vi "LAb4gui.vi"() -> ()   [LabVIEW 2026]
uses:
  Control_Lab4.ctl
  <vilib>/Instr/_visa.llb/VISA Configure Serial Port (Instr).vi
  Serial - Settings.ctl
panel:
  in  "Serial Settings":T1={"baud rate"=115200, "data bits"=8, "parity"=enum."None", "stop bits"=10, "flow control"=0} {"flow control" items=["None"=0, "XON/XOFF"=1, "RTS/CTS"=2, "DTR/DSR"=4]; "stop bits" items=["1.0"=10, "1.5"=15, "2.0"=20]; "data bits" min=5 max=8 step=1; "baud rate" items=["75"=75, "110"=110, "134"=134, "150"=150, "300"=300, "600"=600, "1200"=1200, "1800"=1800, "2400"=2400, "4800"=4800, "7200"=7200, "9600"=9600, "14400"=14400, "19200"=19200, "28800"=28800, "38400"=38400, "56000"=56000, "57600"=57600, "115200"=115200, "128000"=128000, "230400"=230400]}
  in  "Detection Threshold":i32
  in  "stop":bool
  out "Last Command Sent":string
  out "ESP Response":string
  in  "Send Filters":bool
  in  "Blur":dbl(knob) scale=0.0..10.0
  in  "Minimum Area":i32
  in  "Reset Filters":bool
  out "Connected to ESP":bool
  in  "VISA resource name":refnum<visa-resource-name>
  in  "Display ON/OFF":bool
  in  "Get Status":bool
  in  "Identify":bool
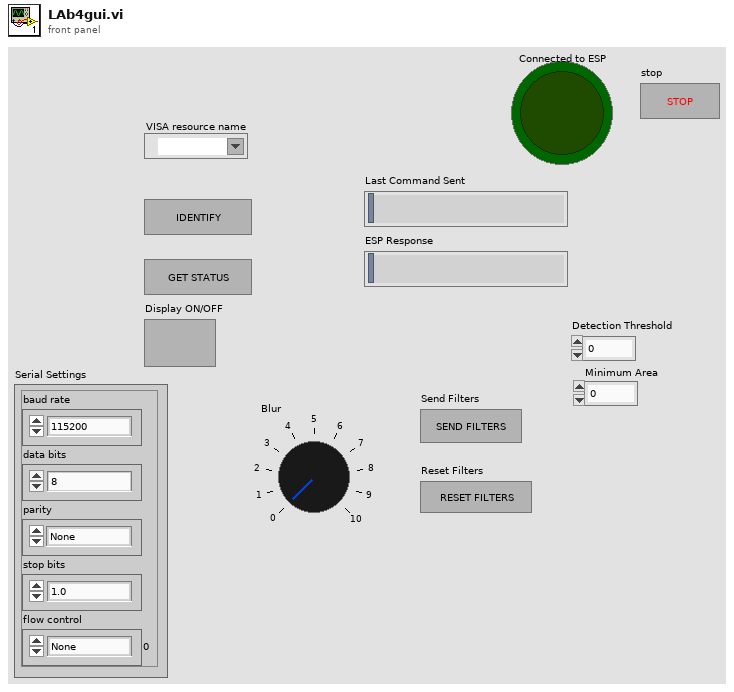
[diagram p1: front panel]
types:
  T1 = typedef "Serial - Settings.ctl" = cluster{"baud rate":u32, "data bits":u16, "parity":enum16{"None", "Odd", "Even", "Mark", "Space"}, "stop bits":u16, "flow control":u16}
  T2 = typedef "Control_Lab4.ctl" = enum16{"Init", "Connect", "Idle", "Get Status", "Display ON", "Display OFF", "Send Filters", "Reset Filters", "Read Reply", "Disconnect", "Error", "Stop"}
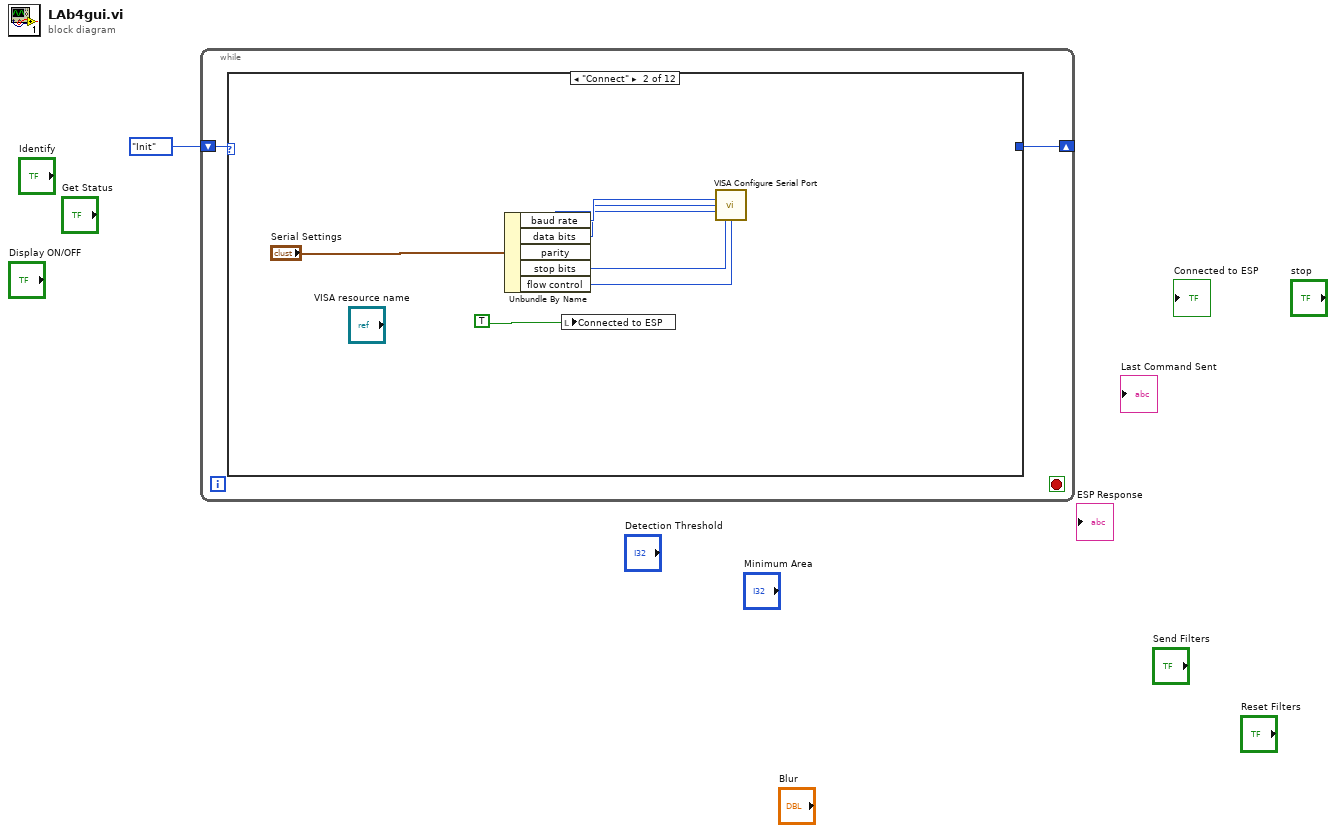
[diagram p0: block diagram]
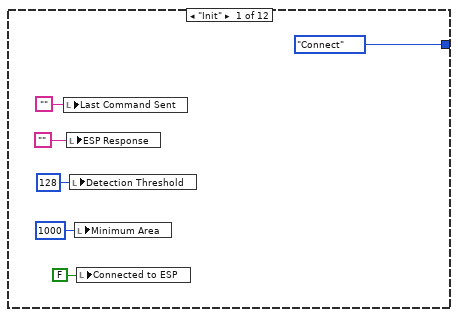
[diagram p2: hidden frame]
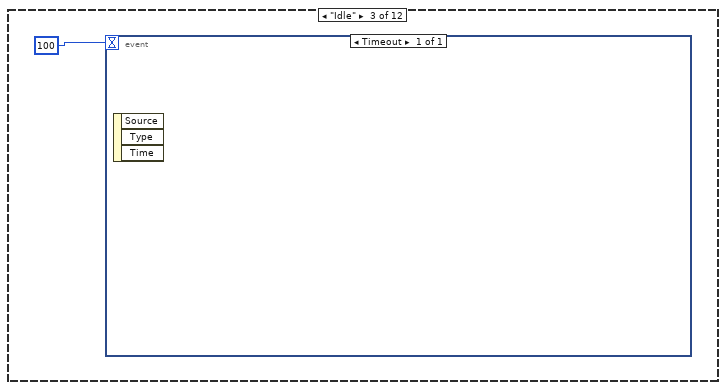
[diagram p3: hidden frame]
diagram:
  n1 = while {
    shift-right: [w2] -> _
    shift-left: Control_Lab4."Init" -> [w3]
    stop <- _ stop-if-true
    n2 = case shown="\"Connect\"" w3 {
      tunnel: [Control_Lab4."Connect" _ _ _ _ _ _ _ _ _ _ _] -> w2
      frame "Init" {
        n3 = local write "Last Command Sent"("") -> ()
        n4 = local write "ESP Response"("") -> ()
        n5 = local write "Detection Threshold"(128 ("Detection Threshold")) -> ()
        n6 = local write "Minimum Area"(1000 ("Minimum Area")) -> ()
        n7 = local write "Connected to ESP"(FALSE ("Connected to ESP")) -> ()
      }
      frame "Connect" {
        n8 = Unbundle By Name("Serial Settings") -> ("baud rate"=w14:u32, "data bits"=w13:u16, "parity"=w12:enum16{"None", "Odd", "Even", "Mark", "Space"}, "stop bits"=w11:u16, "flow control"=w10:u16)
        n9 = local write "Connected to ESP"(TRUE ("Connected to ESP")) -> ()
        n10 = call-poly "VISA Configure Serial Port"("baud rate (9600)"=w14, "data bits (8)"=w13, "parity (0:none)"=w12, "stop bits (10: 1 bit)"=w11, "flow control (0:none)"=w10) -> ()  [unwired: 9 in, 2 out]
      }
      frame "Idle" {
        n11 = event shown="[0] Timeout" {
          selector: _ -> [_]
          dyn-events: _ -> [_]
          timeout: 100 -> [_]
          event Timeout {
            n12 = event-data() -> ()  [unwired: 1 in, 3 out]
          }
        }
      }
      frame "Get Status" {
      }
      frame "Display ON" {
      }
      frame "Display OFF" {
      }
      frame "Send Filters" {
      }
      frame "Reset Filters" {
      }
      frame "Read Reply" {
      }
      frame "Disconnect" {
      }
      frame "Error" {
      }
      frame "Stop" {
      }
    }
  }
